vi "Write Path.vi"(8 "error in (no error)":errorcluster, 10 "Path":path, 11 "Icon in":refnum<class "Icon.lvclass">) -> (0 "error out":errorcluster, 3 "Icon out":refnum<class "Icon.lvclass">)   [LabVIEW 2016, in "Icon.lvclass"]
uses:
  Icon.lvclass
  System.Drawing
  Icon.lvclass/Icon.ctl
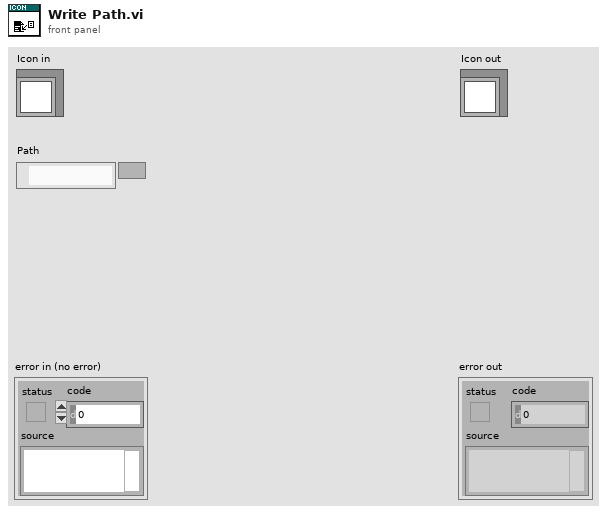
[diagram p1: front panel]
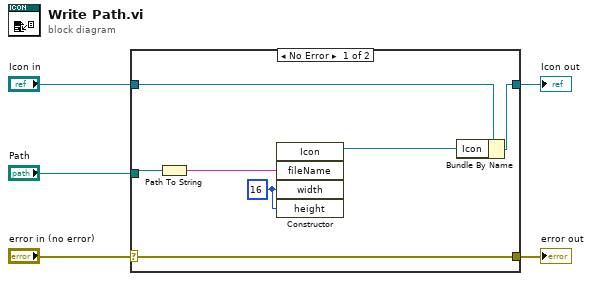
[diagram p0: block diagram]
diagram:
  n1 = case shown="No Error" "error in (no error)" {
    selector: "error in (no error)" -> [w12 w13]
    tunnel: [w12 w13] -> w4
    tunnel: [w11 w14] -> w2
    tunnel: "Icon in" -> [w10 w14]
    tunnel: "Path" -> [w9 _]
    frame No Error {
      w7 = 16 ("width")
      n2 = Path To String(path=w9) -> (string=w8:string)
      n3 = constructor class="Icon"("fileName"=w8, "width"=w7, "height"=w7) -> (reference out=w6:refnum<k24>)  [unwired: 3 in, 5 out]
      n4 = Bundle By Name(cluster=w10, "Icon"=w6) -> (w11:refnum<class "Icon.lvclass">)
    }
    frame Error {
    }
  }
  "error out" <- w4
  "Icon out" <- w2
